vi "test_contrast_map_filtered _M_stripped.vi"() -> ()   [LabVIEW 2009]
doc: "Copyright (C) 2009, Stepan A. Baranov\nweb: http://www.OCTLab.org/\nemail: stepan@baranov.su"
uses:
  <vilib>/Analysis/NI_AALBase.lvlib
  OCTLib.dll
panel:
  out "min":dbl format="%0.2f"
  out "max":dbl format="%0.2f"
  out "offset":i32
  out "error out":errorcluster
  out "strip size":i32
  out "width":i32
  out "height":i32
  in  "Small/Big":bool
  out "loop #":i32
  out "RSM_STAT time":u32
  out "LabView time":u32
  out "RSM_STAT Array":dbl[][](array[numeric])
  out "LabView Array":dbl[][](array[numeric])
  in  "stop":bool
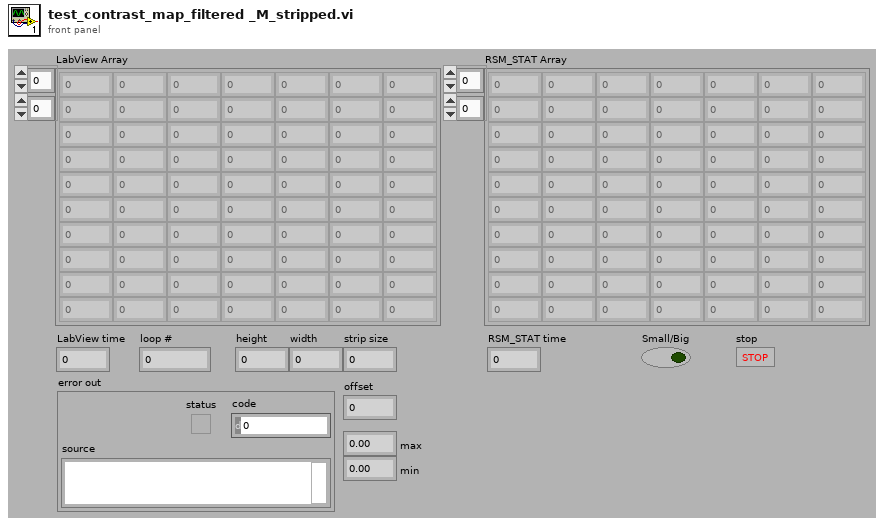
[diagram p1: front panel]
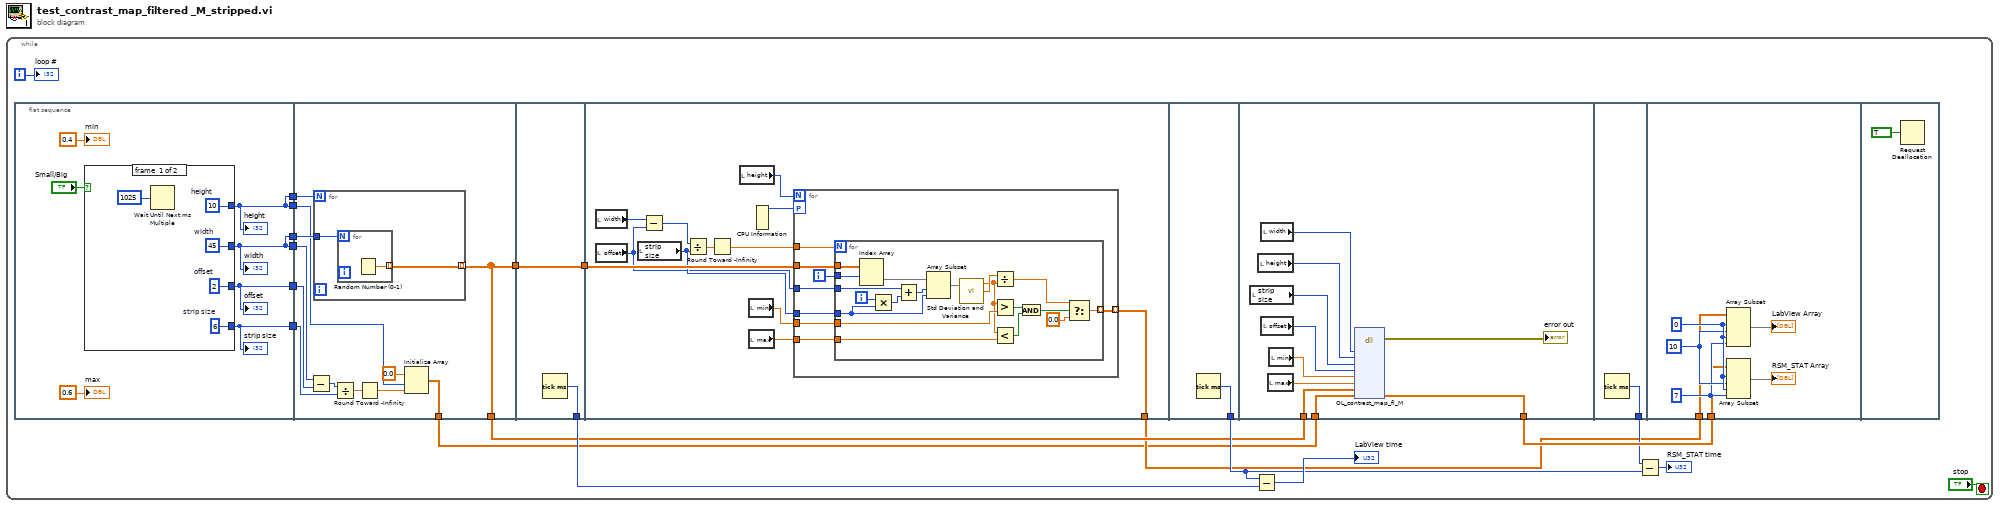
[diagram p0: block diagram]
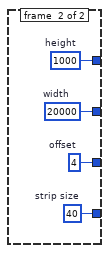
[diagram p2: hidden frame]
diagram:
  n1 = while {
    i -> [w12]
    stop <- "stop" stop-if-true
    n2 = flat-sequence {
      tunnel: [w23] -> w8
      tunnel: [w24] -> w7
      tunnel: [w25] -> w5
      tunnel: [w24] -> w4
      tunnel: [w23] -> w3
      tunnel: [w22] -> w1
      tunnel: [w45] -> w11
      tunnel: [w45] -> w9
      tunnel: w8 -> [w47]
      tunnel: w7 -> [w46]
      tunnel: w5 -> [w38]
      tunnel: w4 -> [w42]
      tunnel: w3 -> [w41]
      tunnel: [w43] -> w2
      tunnel: w1 -> [w40]
      tunnel: [w52] -> w17
      tunnel: [w51] -> w10
      tunnel: w9 -> [w51]
      tunnel: w10 -> [w64]
      tunnel: [w63] -> w6
      tunnel: [w92] -> w14
      tunnel: w11 -> [w101]
      tunnel: [w100] -> w18
      tunnel: w2 -> [w102]
      tunnel: [w103] -> w15
      tunnel: w18 -> [w106]
      tunnel: w6 -> [w105]
      frame #0 {
        n3 = case shown="True" "Small/Big" {
          tunnel: [w29 w35] -> w24
          tunnel: [w30 w34] -> w23
          tunnel: [w31 w33] -> w25
          tunnel: [w27 w32] -> w22
          frame #0 {
            w27 = 2  # offset
            w31 = 6  # strip size
            w30 = 45  # width
            w29 = 10  # height
            n4 = Wait Until Next ms Multiple(millisecond multiple=u32 1025) -> ()  [unwired: 1 out]
          }
          frame #1 {
            w32 = 4  # offset
            w33 = 40  # strip size
            w34 = 20000  # width
            w35 = 1000  # height
          }
        }
        "height" <- w24
        "width" <- w23
        "strip size" <- w25
        "offset" <- w22
        "max" <- 0.6 ("max")
        "min" <- 0.4 ("min")
      }
      frame #1 {
        n5 = Subtract(x=w41, y=w40) -> (x-y=w39:i32)
        n6 = for {
          N: w46 -> [_]
          tunnel: w47 -> [w49]
          tunnel: [w48] -> w45 mode=indexing
          n7 = for {
            N: w49 -> [_]
            tunnel: [w50] -> w48 mode=indexing
            n8 = Random Number (0-1)() -> (number: 0 to 1=w50:dbl)
          }
        }
        n9 = Divide(x=w39, y=w38) -> (x/y=w37:dbl)
        n10 = Round Toward -Infinity(1:w37) -> (0:w36:dbl)
        n11 = Initialize Array(0.0 ("element"), w42, w36) -> (w43:dbl[][])
      }
      frame #2 {
        n12 = Tick Count (ms)() -> (millisecond timer value=w52:u32)
      }
      frame #3 {
        n13 = local read "width"() -> (w62:i32)
        n14 = local read "offset"() -> (w53:i32)
        n15 = local read "strip size"() -> (w56:i32)
        n16 = Subtract(x=w62, y=w53) -> (x-y=w57:i32)
        n17 = Divide(x=w57, y=w56) -> (x/y=w55:dbl)
        n18 = Round Toward -Infinity(1:w55) -> (0:w54:dbl)
        n19 = local read "height"() -> (w58:i32)
        n20 = local read "min"() -> (w60:dbl)
        n21 = local read "max"() -> (w59:dbl)
        n22 = CPU Information() -> (4:w61:i32)  [unwired: 3 out]
        n23 = for {
          N: w58 -> [_]
          tunnel: w64 -> [w71]
          tunnel: [w70] -> w63 mode=indexing
          tunnel: w56 -> [w69]
          tunnel: w54 -> [w68]
          workers-P: w61 -> [_]
          tunnel: w60 -> [w67]
          tunnel: w59 -> [w66]
          tunnel: w53 -> [w65]
          i -> [w72]
          n24 = for {
            N: w68 -> [_]
            tunnel: w72 -> [w77]
            tunnel: w71 -> [w78]
            tunnel: [w84] -> w70 mode=indexing
            tunnel: w69 -> [w74]
            tunnel: w67 -> [w90]
            tunnel: w66 -> [w89]
            tunnel: w65 -> [w79]
            i -> [w81]
            n25 = Index Array(array=w78, index (row)=w77) -> (element=w76:dbl[])  [unwired: 1 in]
            n26 = Multiply(x=w81, y=w74) -> (x*y=w80:i32)
            n27 = Add(x=w79, y=w80) -> (x+y=w75:i32)
            n28 = Array Subset(array=w76, index=w75, length=w74) -> (w73:dbl[])
            n29 = call <vilib>:"Std Deviation and Variance.vi"("X"=w73) -> ("mean"=w82:dbl, "standard deviation"=w91:dbl)  [unwired: 1 in, 1 out]
            n30 = Divide(x=w91, y=w82) -> (x/y=w85:dbl)
            n31 = Greater?(x=w82, y=w90) -> (0:w87:bool)
            n32 = Less?(x=w82, y=w89) -> (x < y?=w88:bool)
            n33 = And(x=w87, y=w88) -> (x .and. y?=w86:bool)
            n34 = Select(t=w85, s=w86, f=0.0) -> (s? t:f=w84:dbl)
          }
        }
      }
      frame #4 {
        n35 = Tick Count (ms)() -> (millisecond timer value=w92:u32)
      }
      frame #5 {
        n36 = local read "strip size"() -> (w96:i32)
        n37 = local read "height"() -> (w98:i32)
        n38 = local read "width"() -> (w99:i32)
        n39 = local read "offset"() -> (w95:i32)
        n40 = local read "max"() -> (w93:dbl)
        n41 = local read "min"() -> (w94:dbl)
        n42 = dll-call lib="OCTLib.dll" fn="OL_contrast_map_fl_M"("width"=w99, "height"=w98, "stripsize"=w96, "offset"=w95, "min"=w94, "max"=w93, "input"=w101, "output"=w102) -> (error out=→"error out":errorcluster, "output"=w100:dbl[][])  [unwired: 11 in, 1 out]
      }
      frame #6 {
        n43 = Tick Count (ms)() -> (millisecond timer value=w103:u32)
      }
      frame #7 {
        w109 = 10 ("length")
        w108 = 7 ("length")
        w110 = 0 ("index")
        n44 = Array Subset(array=w105, index (row)=w110, length (row)=w109, index (col)=w110, length (col)=w108) -> (→"LabView Array":dbl[][])
        n45 = Array Subset(array=w106, index (row)=w110, length (row)=w109, index (col)=w110, length (col)=w108) -> (→"RSM_STAT Array":dbl[][])
      }
      frame #8 {
        n46 = Request Deallocation(TRUE ("flag")) -> ()
      }
    }
    n47 = Subtract(x=w14, y=w17) -> (x-y=→"LabView time":u32)
    n48 = Subtract(x=w15, y=w14) -> (x-y=→"RSM_STAT time":u32)
    "loop #" <- w12
  }
